vi "DSF.Shared.Configuration.Framework.Get All Transfer Configurations.vi"(8 "error in (no error)":errorcluster, 11 "Framework Configuration in":refnum<class "DSF.Shared.Configuration.Framework.lvclass">) -> (0 "error out":errorcluster, 2 "Transfer Configurations":T1[](array[typedef]), 3 "Framework Configuration out":refnum<class "DSF.Shared.Configuration.Framework.lvclass">)   [LabVIEW 2017, in "DSF.Engine.lvlib" / "DSF.Shared.Configuration.Framework.lvclass"]
uses:
  DSF.Shared.Configuration.Framework.lvclass
  Typedefs/DSF.Shared.Refactor.Typedefs.Transfer Configuration.ctl
  Typedefs/DSF.Shared.Typedefs.Byte Order.ctl
  Typedefs/DSF.Shared.Refactor.Typedefs.Channel Array Configuration.ctl
  Typedefs/DSF.Shared.Typedefs.Data Type.ctl
  DSF.Shared.Configuration.Framework.lvclass/DSF.Shared.Configuration.Framework.ctl
  DSF.Engine.lvlib
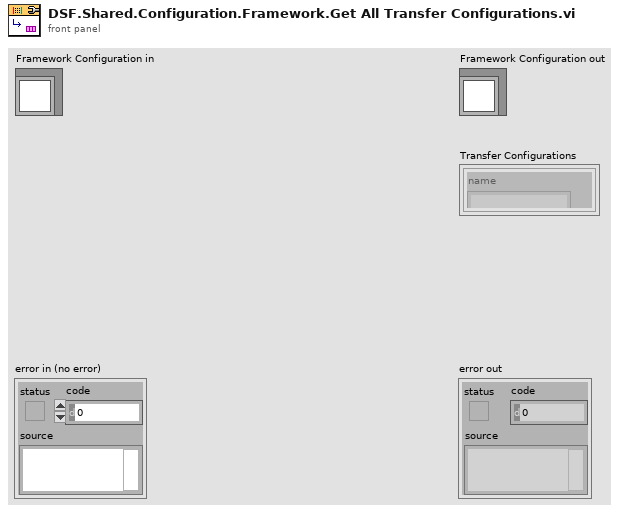
[diagram p1: front panel]
types:
  T1 = typedef "DSF.Engine.lvlib/DSF.Shared.Refactor.Typedefs.Transfer Configuration.ctl" = cluster{"name":string, "byte order":T2, "channel configurations":T3[]}
  T2 = typedef "DSF.Engine.lvlib/DSF.Shared.Typedefs.Byte Order.ctl" = enum8{"big-endian", "little-endian"}
  T3 = typedef "DSF.Engine.lvlib/DSF.Shared.Refactor.Typedefs.Channel Array Configuration.ctl" = cluster{"name":string, "data type":T4, "count":u64, "buffer offset":u64, "engine offset":u64}
  T4 = typedef "DSF.Engine.lvlib/DSF.Shared.Typedefs.Data Type.ctl" = enum8{"Bool", "SGL", "DBL", "I8", "I16", "I32", "I64", "U8", "U16", "U32", "U64"}
  T5 = typedef "DSF.Engine.lvlib/DSF.Shared.Refactor.Typedefs.Framework Configuration.Aggregate.ctl" = cluster{"Plugins":T6[]}
  T6 = typedef "DSF.Engine.lvlib/DSF.Shared.Refactor.Typedefs.Plugin Configuration.Aggregate.ctl" = cluster{"name":string, "class":string, "cycle timing":T7, "Transfer Groups":T8[]}
  T7 = typedef "DSF.Engine.lvlib/DSF.Shared.Typedefs.Cycle Timing Factors.ctl" = cluster{"Priority":u64, "Decimation":u64, "Offset":u64}
  T8 = typedef "DSF.Engine.lvlib/DSF.Shared.Refactor.Typedefs.Transfer Group Configuration.Aggregate.ctl" = cluster{"name":string, "direction":T9, "cycle timing":T7, "Transfers":T1[]}
  T9 = typedef "DSF.Engine.lvlib/DSF.Shared.Typedefs.Direction.ctl" = enum8{"Tx", "Rx"}
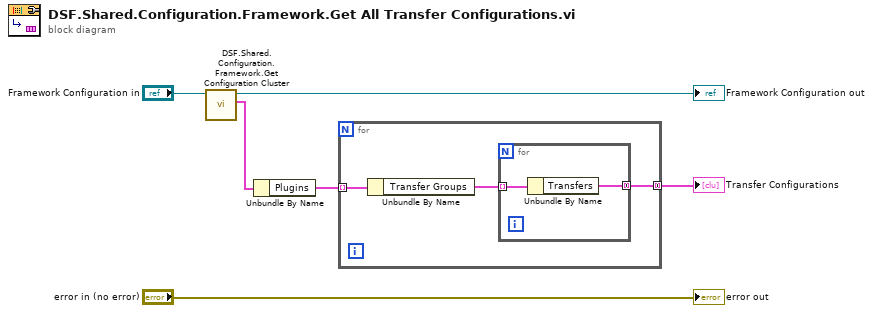
[diagram p0: block diagram]
diagram:
  n1 = call "DSF.Shared.Configuration.Framework.Get Configuration Cluster.vi"("Framework Configuration in"="Framework Configuration in") -> ("Framework Configuration"=w1:T5, "Framework Configuration out"=→"Framework Configuration out":refnum<class "DSF.Shared.Configuration.Framework.lvclass">)  [unwired: 9 in]
  n2 = Unbundle By Name(w1) -> ("Plugins"=w5:T6[])
  n3 = for {
    tunnel: w5 -> [w9] mode=indexing
    tunnel: [w7] -> w4 mode=concatenating
    n4 = Unbundle By Name(w9) -> ("Transfer Groups"=w8:T8[])
    n5 = for {
      tunnel: w8 -> [w11] mode=indexing
      tunnel: [w10] -> w7 mode=concatenating
      n6 = Unbundle By Name(w11) -> ("Transfers"=w10:T1[])
    }
  }
  "Transfer Configurations" <- w4
  "error out" <- "error in (no error)"
